vi "TxPkt - Add Packet.vi"(5 "Add Port Channel":bool, 8 "error in (no error)":errorcluster, 9 "New Packet ID":i32, 10 "New Packet Name":string, 11 "Item Ref in":T1=18446744073709551615 format="%.0x") -> (0 "error out":errorcluster, 2 "New Packet Ref":T1=18446744073709551615 format="%.0x", 3 "Item Ref Out":T1=18446744073709551615 format="%.0x")   [LabVIEW 2019, in "UDP-Custom-Device System Explorer.lvlib"]
uses:
  UDP-Custom-Device System Explorer.lvlib
  <vilib>/NI VeriStand/Custom Device API/Custom Device Item Ref.ctl
  Shared/Constants.vi
  Shared/UDP-Custom-Device Shared.lvlib
  <vilib>/NI VeriStand/Custom Device API/Custom Device API.lvlib
  Property Accessors/Shared Section Accessors.lvlib
  Property Accessors/Shared Packet Accessors.lvlib
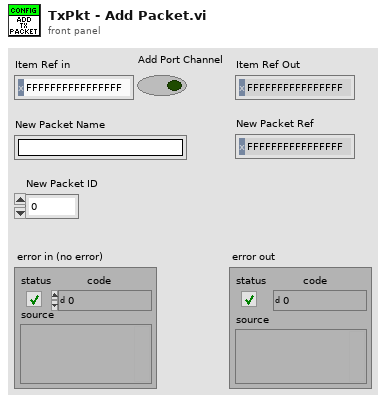
[diagram p1: front panel]
types:
  T1 = typedef "Custom Device API.lvlib/Custom Device Item Ref.ctl" = u64
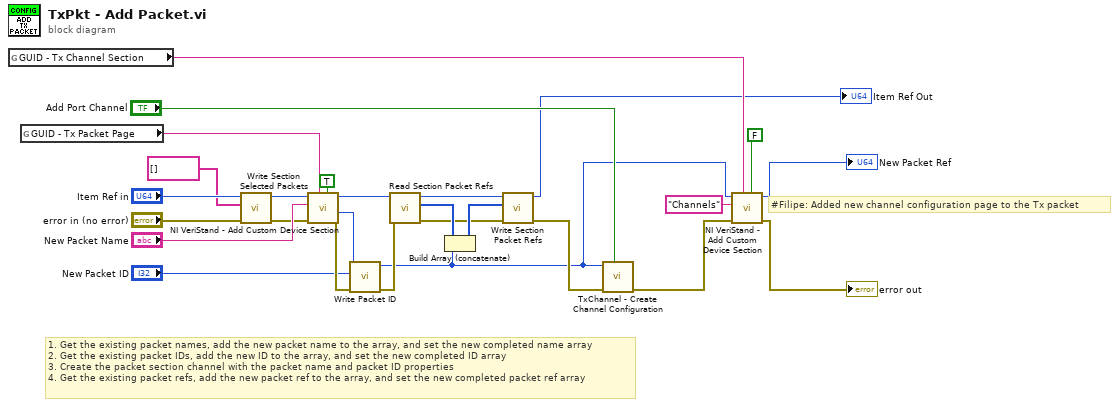
[diagram p0: block diagram]
diagram:
  # "#Filipe: Added new channel configuration page to the Tx packet"
  # "1. Get the existing packet names, add the new packet name to the array, and set the new completed name array\n2. Get the existing packet IDs, add the new ID to the array, and set the new completed ID array\n3. Create the packet section channel with the packet name and packet ID properties\n4. Get the existing packet refs, add the new packet ref to the array, and set the new completed packet ref array"
  n1 = global read "Constants.vi" "GUID - Tx Channel Section"() -> (w6:string)
  n2 = global read "Constants.vi" "GUID - Tx Packet Page"() -> (w26:string)
  n3 = call "Write Section Selected Packets.vi"("error in (no error)"="error in (no error)", "Selected Packets"=string[] [] ("Value"), "Node Ptr"="Item Ref in") -> ("error out"=w16:errorcluster, "Node Ptr out"=w15:T1)  [unwired: 7 in]
  n4 = call <vilib>:"NI VeriStand - Add Custom Device Section.vi"("Highlight? (F)"=TRUE, "GUID (Default Section)"=w26, "error in (no error)"=w16, "Section Name"="New Packet Name", "Parent Ref in"=w15) -> ("error out"=w12:errorcluster, "Section Ptr"=w13:T1, "Parent Ref out"=w24:T1)  [unwired: 3 in, 1 out]
  n5 = call "Write Packet ID.vi"("error in (no error)"=w12, "Packet ID"="New Packet ID", "Node Ptr"=w13) -> ("error out"=w11:errorcluster, "Node Ptr out"=w2:T1)  [unwired: 7 in]
  n6 = call "Read Section Packet Refs.vi"("error in (no error)"=w11, "Node Ptr"=w24) -> ("error out"=w20:errorcluster, "Dependent Node Refs"=w22:T1[], "Node Ptr out"=w23:T1)  [unwired: 7 in]
  n7 = Build Array (concatenate)(w22, w2) -> (w21:T1[])
  n8 = call "Write Section Packet Refs.vi"("error in (no error)"=w20, "Dependent Node Refs"=w21, "Node Ptr"=w23) -> ("error out"=w19:errorcluster, "Node Ptr out"=→"Item Ref Out":T1)  [unwired: 7 in]
  n9 = call "TxChannel - Create Channel Configuration.vi"("Add Port Channel"="Add Port Channel", "error in (no error)"=w19, "Parent Packet Ref"=w2) -> ("error out"=w8:errorcluster)  [unwired: 7 in, 1 out]
  n10 = call <vilib>:"NI VeriStand - Add Custom Device Section.vi"("Highlight? (F)"=FALSE, "GUID (Default Section)"=w6, "error in (no error)"=w8, "Section Name"="Channels", "Parent Ref in"=w2) -> ("error out"=→"error out":errorcluster, "Parent Ref out"=→"New Packet Ref":T1)  [unwired: 3 in, 2 out]
